vi "Boiler Controller.vi"(8 "Error In":errorcluster, 11 "Message Queues":T1) -> (0 "Error Out":errorcluster)   [LabVIEW 2015]
uses:
  support/Message Queue/All Message Queues.ctl
  support/Message Queue/Message Cluster.ctl
  support/Message Queue/Message Queue.lvlib
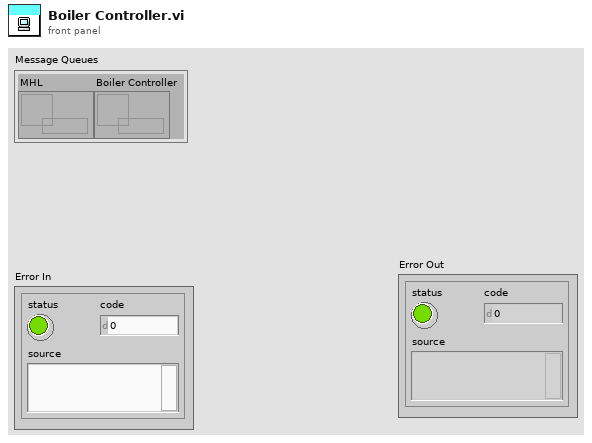
[diagram p1: front panel]
types:
  T1 = typedef "Message Queue.lvlib/All Message Queues.ctl" = cluster{"MHL":refnum<queue>, "Boiler Controller":refnum<queue>}
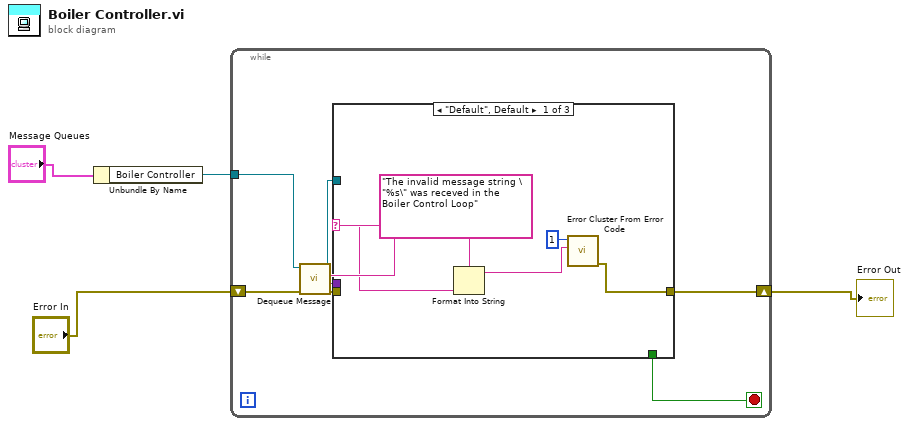
[diagram p0: block diagram]
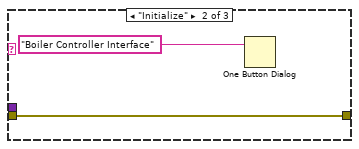
[diagram p2: hidden frame]
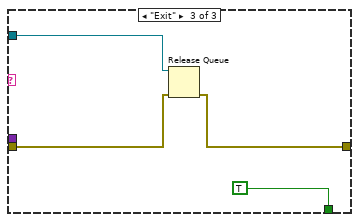
[diagram p3: hidden frame]
diagram:
  n1 = Unbundle By Name("Message Queues") -> ("Boiler Controller"=w3:refnum<queue>)
  n2 = while {
    tunnel: w3 -> [w12]
    shift-right: [w6] -> w1
    shift-left: "Error In" -> [w11]
    stop <- w5 stop-if-true
    n3 = call "Dequeue Message.vi"("error in (no error)"=w11, "Message Queue"=w12) -> ("error out"=w8:errorcluster, "Message Data"=w7:variant, "Message"=w10:string, "dup Message Queue"=w9:refnum<queue>)  [unwired: 6 in]
    n4 = case shown="\"Default\", Default" w10 {
      selector: w10 -> [w13 _ _]
      tunnel: w9 -> [_ _ w23]
      tunnel: w8 -> [_ w18 w22]
      tunnel: w7 -> [_ _ _]
      tunnel: [w16 w18 w21] -> w6
      tunnel: [_ _ TRUE] -> w5
      frame "Default", Default {
        n5 = Format Into String(format string="The invalid message string \"%s\" was receved in the Boiler Control Loop", w13) -> (resulting string=w14:string)  [unwired: 2 in, 1 out]
        n6 = call <vilib>:"Error Cluster From Error Code.vi"("error message (\"\")"=w14, "error code (0)"=1) -> ("error out"=w16:errorcluster)  [unwired: 7 in]
      }
      frame "Initialize" {
        n7 = One Button Dialog(message="Boiler Controller Interface") -> ()  [unwired: 1 in, 1 out]
      }
      frame "Exit" {
        n8 = Release Queue(queue=w23, error in (no error)=w22) -> (error out=w21:errorcluster)  [unwired: 1 in, 2 out]
      }
    }
  }
  "Error Out" <- w1
